vi "Counter - Read Encoder (Finite Clock).vi"() -> ()   [LabVIEW 2022 SP3]
doc: "This example demonstrates how to acquire a finite buffer of encoder measurements using a DAQmx device. It uses an external clock so that the samples of the count register occur at regular intervals. If you do not need deterministic sampling of the count register, refer instead to the Counter - Read Encoder.vi example which does not use an external clock.\n\nFor instructions on how to connect your signals to the DAQ device, refer to your device documentation."
uses:
  <vilib>/Utility/error.llb/DialogType.ctl
  <vilib>/DAQmx/read.llb/DAQmx Read (Counter 1D DBL 1Chan NSamp).vi
  <vilib>/DAQmx/create/channels.llb/DAQmx Create Channel (CI-Position-Angular Encoder).vi
  <vilib>/DAQmx/configure/timing.llb/DAQmx Timing (Sample Clock).vi
  <vilib>/DAQmx/miscellaneous.llb/DAQmx Fill In Error Info.vi
  <resource>/objmgr/daqmx.rc
panel:
  in  "Z Index Terminal":tag="PFI9"
  in  "Z Index Enable":bool
  in  "Pulses Per Revolution":u32=24
  in  "B Input Terminal":tag="PFI10"
  in  "A Input Terminal":tag="PFI8"
  in  "Counter":tag="Dev1/ctr0"
  in  "Trigger Type":enum32{"No Trigger", "Digital Arm Start"}(tab)
  in  "Edge":i32(ring)=10280 items=["Rising"=10280, "Falling"=10171]
  in  "Digital Trigger Source":tag
  out "Acquired Data":dbl[](array[numeric])
  in  "Samples":i32=100
  in  "Sample Rate":dbl=1000.0
  in  "Sample Clock Source":tag="PFI0"
  # "Channel Settings"
  # "Acquired Data"
  # "Timing Settings"
  # "Trigger Settings"
  # "To configure and use a trigger or the count reset you must have the necessary tab selected above.  Not all hardware supports the above options--refer to your device documentation for more info."
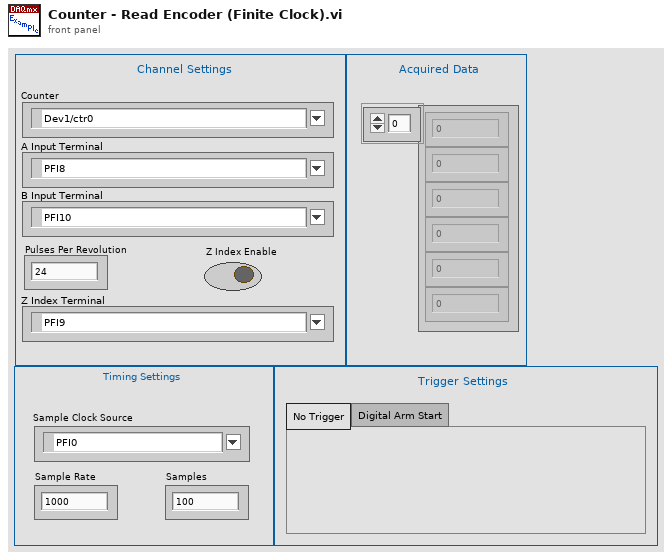
[diagram p1: front panel]
types:
  T1 = typedef "DialogType.ctl" = u16
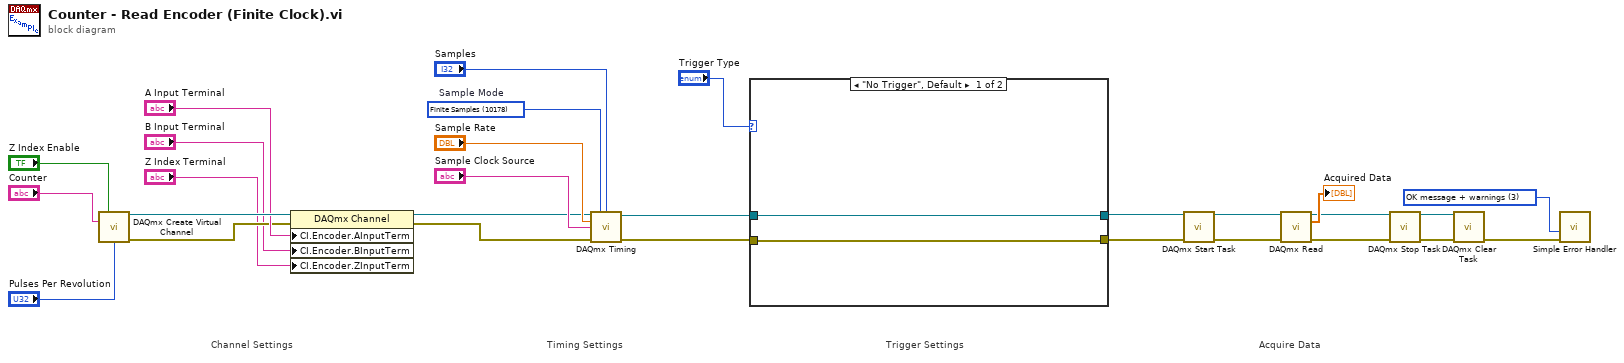
[diagram p0: block diagram]
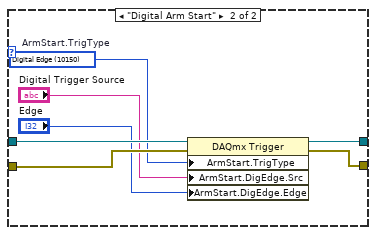
[diagram p2: hidden frame]
diagram:
  w1 = T1 3 items=["no dialog", "OK message", "continue or stop message", "OK message + warnings", "continue/stop + warnings"] ("type of dialog (OK msg:1)")
  w28 = 10178 items=["Finite Samples"=10178, "Continuous Samples"=10123, "Hardware Timed Single Point"=12522]  # Sample Mode
  # "Acquire Data"
  # "Trigger Settings"
  # "Timing Settings"
  # "Channel Settings"
  n1 = call-poly <vilib>:"DAQmx Create Virtual Channel.vi"("z index enable"="Z Index Enable", "counter"="Counter", "pulses per revolution"="Pulses Per Revolution") -> ("task out"=w14:refnum<k21>, "error out"=w12:errorcluster)  [unwired: 11 in]
  n2 = property class="DAQmx Channel"(reference=w14, error in=w12, "CI.Encoder.AInputTerm"="A Input Terminal", "CI.Encoder.BInputTerm"="B Input Terminal", "CI.Encoder.ZInputTerm"="Z Index Terminal") -> (reference out=w7:refnum<k21>, error out=w6:errorcluster)
  n3 = call-poly <vilib>:"DAQmx Timing.vi"("task/channels in"=w7, "sample mode"=w28, "samples per channel"="Samples", "rate"="Sample Rate", "source"="Sample Clock Source", "error in"=w6) -> ("task out"=w18:refnum<k21>, "error out"=w19:errorcluster)  [unwired: 8 in]
  n4 = case shown="\"No Trigger\", Default" "Trigger Type" {
    tunnel: w18 -> [w30 w37]
    tunnel: w19 -> [w29 w34]
    tunnel: [w30 w36] -> w16
    tunnel: [w29 w35] -> w17
    frame "No Trigger", Default {
    }
    frame "Digital Arm Start" {
      w31 = 10150 items=["Digital Edge"=10150, "None"=10230]  # ArmStart.TrigType
      n5 = property class="DAQmx Trigger"(reference=w37, error in=w34, "ArmStart.TrigType"=w31, "ArmStart.DigEdge.Src"="Digital Trigger Source", "ArmStart.DigEdge.Edge"="Edge") -> (reference out=w36:refnum<k21>, error out=w35:errorcluster)
    }
  }
  n6 = call <vilib>:"DAQmx Start Task.vi"("task/channels in"=w16, "error in"=w17) -> ("task out"=w27:refnum<k21>, "error out"=w26:errorcluster)  [unwired: 12 in]
  n7 = call-poly <vilib>:"DAQmx Read.vi"("task/channels in"=w27, "error in"=w26) -> ("task out"=w2:refnum<k21>, "data"=→"Acquired Data":dbl[], "error out"=w3:errorcluster)  [unwired: 11 in]
  n8 = call <vilib>:"DAQmx Stop Task.vi"("task/channels in"=w2, "error in"=w3) -> ("task out"=w4:refnum<k21>, "error out"=w5:errorcluster)  [unwired: 12 in]
  n9 = call <vilib>:"DAQmx Clear Task.vi"("task in"=w4, "error in"=w5) -> ("error out"=w25:errorcluster)  [unwired: 13 in]
  n10 = call <vilib>:"Simple Error Handler.vi"("type of dialog (OK msg:1)"=w1, "error in (no error)"=w25) -> ()  [unwired: 3 in, 5 out]
